vi "MetaSaveToInfoFile.vi"(8 "error in (no error)":errorcluster, 11 "File Paths":T1={"Local Save Path"=path "\\\\smbhome.uscs.susx.ac.uk\\cv222/Desktop/data", "Newton Save Path"=path "Z:/#Projects/Entanglement/data", "File Name"="test", "LocalSave"=TRUE}) -> (0 "error out":errorcluster)   [LabVIEW 2017]
uses:
  controls/FilePaths.ctl
  controls/GlobalExp.vi
  Global.lvlib
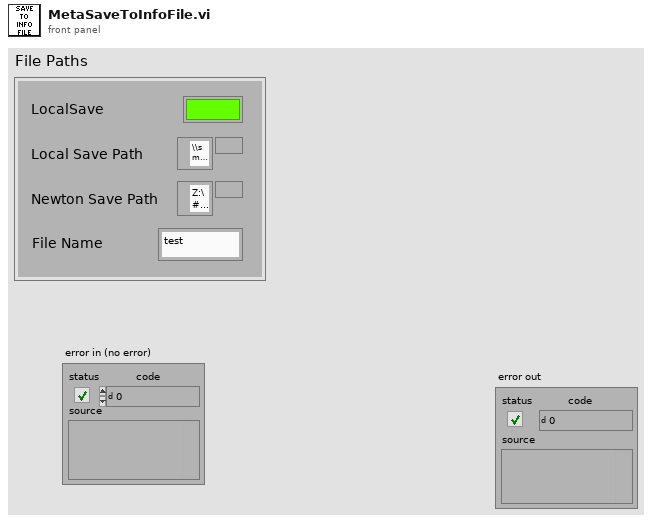
[diagram p1: front panel]
types:
  T1 = typedef "FilePaths.ctl" = cluster{"Local Save Path":path, "Newton Save Path":path, "File Name":string, "LocalSave":bool}
  T2 = cluster{"ExpNum":i32, "ExpParams":cluster{"ExpName":string, "Det":i32, "Step":i32, "state":string, "freq":i32, "amp":i32}}
  T3 = enum16{"open", "replace", "create", "open or create", "replace or create", "replace or create with confirmation"}
  T4 = typedef "MasterExpControl.ctl" = cluster{"Main Steps":dbl, "Main Runs":dbl, "ExpStatus":enum16{"Innit", "Stop", "Idle", "MainRunning", "AuxRunning"}, "Main Current Step":dbl, "ExpNum":dbl, "NewData":bool, "date":string, "command":string, "Stop":bool, "Pause":bool, "Mathematica":string, "Main/Meta":bool, "UpdateMath":bool, "Camera":bool}
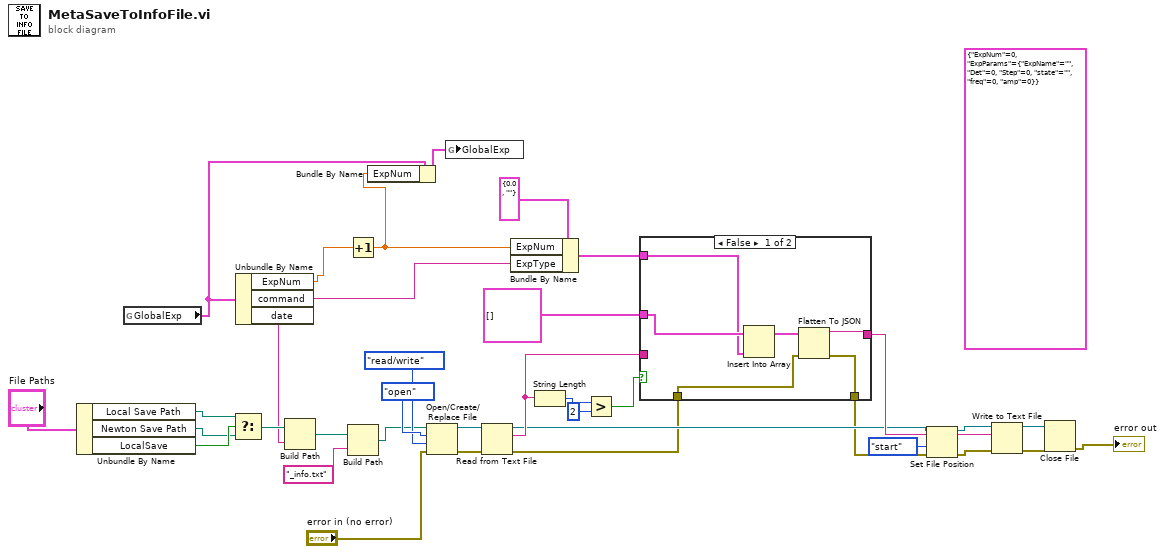
[diagram p0: block diagram]
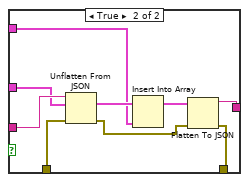
[diagram p2: hidden frame]
diagram:
  (unwired) T2 {"ExpNum"=0, "ExpParams"={"ExpName"="", "Det"=0, "Step"=0, "state"="", "freq"=0, "amp"=0}}
  n1 = Unbundle By Name("File Paths") -> ("Local Save Path"=w34:path, "Newton Save Path"=w33:path, "LocalSave"=w35:bool)
  n2 = global read "GlobalExp.vi" "GlobalExp"() -> (w8:T4)
  n3 = Select(t=w34, s=w35, f=w33) -> (s? t:f=w32:path)
  n4 = Unbundle By Name(w8) -> ("ExpNum"=w10:dbl, "command"=w19:string, "date"=w31:string)
  n5 = Build Path(base path=w32, name or relative path=w31) -> (appended path=w13:path)
  n6 = Increment(x=w10) -> (x+1=w7:dbl)
  n7 = Build Path(base path=w13, name or relative path="_info.txt") -> (appended path=w11:path)
  n8 = Bundle By Name(cluster=w8, "ExpNum"=w7) -> (w9:T4)
  n9 = Open/Create/Replace File(file path (use dialog)=w11, error in="error in (no error)", operation (0:open)=T3."open", access (0:read/write)=enum16{"read/write", "read-only", "write-only"}."read/write") -> (refnum out=w28:refnum<file>, error out=w27:errorcluster)  [unwired: 2 in, 1 out]
  n10 = global write "GlobalExp.vi" "GlobalExp"(w9) -> ()
  n11 = Read from Text File(file (use dialog)=w28, error in=w27) -> (refnum out=w4:refnum<file>, text=w23:string, error out=w3:errorcluster)  [unwired: 2 in, 1 out]
  n12 = Bundle By Name(cluster=cluster{"ExpNum":dbl, "ExpType":string} {"ExpNum"=0.0, "ExpType"=""} ("Cluster"), "ExpNum"=w7, "ExpType"=w19) -> (w18:cluster{"ExpNum":dbl, "ExpType":string})
  n13 = String Length(string=w23) -> (length=w26:i32)
  n14 = Greater?(x=w26, y=2) -> (0:w24:bool)
  n15 = case shown="False" w24 {
    tunnel: w23 -> [_ w51]
    tunnel: cluster{"ExpNum":dbl, "ExpType":string}[] [] ("InfoFile") -> [w40 w50]
    tunnel: w18 -> [w39 w48]
    tunnel: [w41 w46] -> w17
    tunnel: w3 -> [w38 w45]
    tunnel: [w37 w43] -> w2
    frame False {
      n16 = Insert Into Array(array=w40, new element=w39) -> (w42:cluster{"ExpNum":dbl, "ExpType":string}[])  [unwired: 1 in]
      n17 = Flatten To JSON(anything=w42, error in (no error)=w38) -> (JSON string=w41:string, 11:w37:errorcluster)  [unwired: 1 in]
    }
    frame True {
      n18 = Unflatten From JSON(JSON string=w51, type and defaults=w50, error in (no error)=w45) -> (value=w49:cluster{"ExpNum":dbl, "ExpType":string}[], error out=w44:errorcluster)  [unwired: 4 in]
      n19 = Insert Into Array(array=w49, new element=w48) -> (w47:cluster{"ExpNum":dbl, "ExpType":string}[])  [unwired: 1 in]
      n20 = Flatten To JSON(anything=w47, error in (no error)=w44) -> (JSON string=w46:string, 11:w43:errorcluster)  [unwired: 1 in]
    }
  }
  n21 = Set File Position(refnum=w4, from (0:start)=enum16{"start", "end", "current"}."start", error in=w2) -> (refnum out=w5:refnum<file>, error out=w6:errorcluster)  [unwired: 1 in]
  n22 = Write to Text File(file (use dialog)=w5, text=w17, error in=w6) -> (refnum out=w15:refnum<file>, error out=w16:errorcluster)  [unwired: 1 in, 1 out]
  n23 = Close File(refnum=w15, error in=w16) -> (error out=→"error out":errorcluster)  [unwired: 1 out]
